vi "JSON Config With Single Term Unit Tests.vi"(8 "error in (no error)":errorcluster) -> (0 "error out":errorcluster)   [LabVIEW 2021]
uses:
  Source/Abs_Types/Double Float/Abs_Double Float.lvclass
  C:/New folder/LV_Abstract/LV_Abstract/Source/Abs_Types/Type/Abs_Type.lvclass
  Source/Abs_Types/Extended Float/Abs_Extended Float.lvclass
  Source/Abs_Types/Single Float/Abs_Single Float.lvclass
  Source/Abs_Types/Time/Abs_Time.lvclass
  Source/Abs_Types/I8 Integer/Abs_I8 Integer.lvclass
  Source/Abs_Types/I16 Integer/Abs_I16 Integer.lvclass
  Source/Abs_Types/I32 Integer/Abs_I32 Integer.lvclass
  Source/Abs_Types/I64 Integer/Abs_I64 Integer.lvclass
  Source/Abs_Types/U8 Integer/Abs_U8 Integer.lvclass
  Source/Abs_Types/U16 Integer/Abs_U16 Integer.lvclass
  Source/Abs_Types/U32 Integer/Abs_U32 Integer.lvclass
  Source/Abs_Types/U64 Integer/Abs_U64 Integer.lvclass
  Source/Abs_Types/Boolean/Abs_Boolean.lvclass
  <vilib>/numeric/Random Number (Range) DBL.vi
  bccc286b-51a7-469e-8471-aa6067be8b2c.vi
  0185a0b0-9277-4e68-a1e4-b3c67cfca5c7.vi
  39d0dc4a-455a-47ed-a8e3-229f4b41d81c.vi
  0d6305d3-07e6-45b2-bcbf-3ecd85e39c77.vi
  e5a5c62c-83b1-472a-b9f7-800ccf0aa222.vi
  cbc5ad68-3937-4771-b877-ea089d07db10.vi
  93f263c1-edcd-4840-9fac-131b8943a342.vi
  5734def3-2dae-4731-9c4b-9a8b4cb92b39.vi
  058e2dda-ae8c-4110-a64d-50d301148ec2.vi
  621c1d66-53be-4b89-8b9b-a8da23b97684.vi
  5add5537-167c-4ec9-aaa0-2258df0f0cfb.vi
  Source/Abs_Types/Abs_Simple_Read.vi
  Source/Abs_Types/Boolean/Simple Read.vi
  Source/Abs_Types/Double Float/Simple Read.vi
  Source/Abs_Types/Extended Float/Simple Read.vi
  Source/Abs_Types/Single Float/Simple Read.vi
  Source/Abs_Types/I8 Integer/Simple Read.vi
  Source/Abs_Types/I16 Integer/Simple Read.vi
  Source/Abs_Types/I32 Integer/Simple Read.vi
  Source/Abs_Types/I64 Integer/Simple Read.vi
  Source/Abs_Types/U8 Integer/Simple Read.vi
  Source/Abs_Types/U16 Integer/Simple Read.vi
  Source/Abs_Types/U32 Integer/Simple Read.vi
  Source/Abs_Types/U64 Integer/Simple Read.vi
  Source/Constants/Support/DBL/Const_DBL.lvclass
  C:/New folder/LV_Abstract/LV_Abstract/Source/Abs_Types/Double Float/Abs_Double Float.lvclass
  Source/Constants/Support/U8/Const_U8.lvclass
  C:/New folder/LV_Abstract/LV_Abstract/Source/Abs_Types/U8 Integer/Abs_U8 Integer.lvclass
  Source/Constants/Support/U16/Const_U16.lvclass
  C:/New folder/LV_Abstract/LV_Abstract/Source/Abs_Types/U16 Integer/Abs_U16 Integer.lvclass
  Source/Constants/Support/U32/Const_U32.lvclass
  C:/New folder/LV_Abstract/LV_Abstract/Source/Abs_Types/U32 Integer/Abs_U32 Integer.lvclass
  Source/Constants/Support/U64/Const_U64.lvclass
  C:/New folder/LV_Abstract/LV_Abstract/Source/Abs_Types/U64 Integer/Abs_U64 Integer.lvclass
  <vilib>/Utility/Data Type/Get Type Information.vi
  Source/Constants/Abs_Constant.vi
  Source/Constants/Support/Bool/Bool.vi
  Source/Functions/Logic/NOT.vi
  Source/Functions/Logic/Support/NOT/Bool/Method.vi
  <vilib>/addons/_JKI Toolkits/Caraya/classes/Test/Define Test.vi
  Source/Abs_Types/Type/Read Config JSON.vi
  <vilib>/addons/_JKI Toolkits/Caraya/classes/Assert/Assert.vi
  <vilib>/addons/_JKI Toolkits/Caraya/classes/Assert/Assert Equal Value_Variant.vi
  <vilib>/addons/_JKI Toolkits/Caraya/classes/Assert/Assert Equal Type_Variant.vi
  Source/Constants/Support/DBL/DBL.vi
  Source/Functions/Math/Increment.vi
  Source/Functions/Math/Support/Increment/DBL/Method.vi
  <vilib>/addons/_JKI Toolkits/Caraya/classes/Assert/Assert Almost Equal_Float.vi
  Source/Constants/Support/EXT/EXT.vi
  Source/Functions/Math/Support/Increment/EXT/Method.vi
  Source/Constants/Support/SGL/SGL.vi
  Source/Functions/Math/Support/Increment/SGL/Method.vi
  Source/Constants/Support/I8/I8.vi
  Source/Functions/Math/Support/Increment/I8/Method.vi
  Source/Constants/Support/I16/I16.vi
  Source/Functions/Math/Support/Increment/I16/Method.vi
  Source/Constants/Support/I32/I32.vi
  Source/Functions/Math/Support/Increment/I32/Method.vi
  Source/Constants/Support/I64/I64.vi
  Source/Functions/Math/Support/Increment/I64/Method.vi
  Source/Constants/Support/U8/U8.vi
  Source/Functions/Math/Support/Increment/U8/Method.vi
  Source/Constants/Support/U16/U16.vi
  Source/Functions/Math/Support/Increment/U16/Method.vi
  Source/Constants/Support/U32/U32.vi
  Source/Functions/Math/Support/Increment/U32/Method.vi
  Source/Constants/Support/U64/U64.vi
  Source/Functions/Math/Support/Increment/U64/Method.vi
  Source/Abs_Types/String/Abs_String.lvclass
  Source/Abs_Types/Complex Double Float/Abs_Complex Double Float.lvclass
  Source/Abs_Types/Complex Extended Float/Abs_Complex Extended Float.lvclass
  Source/Abs_Types/Complex Single Float/Abs_Complex Single Float.lvclass
  18c1a2b9-ea50-4f09-a971-12eb1851eb62.vi
  244b6114-7487-4987-886a-4a2847255e45.vi
  dd58c806-1dee-4031-903d-f938dbea0657.vi
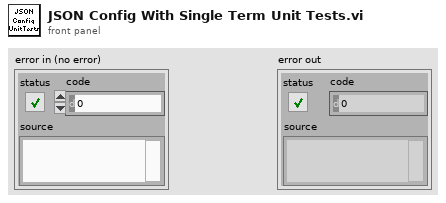
[diagram p1: front panel]
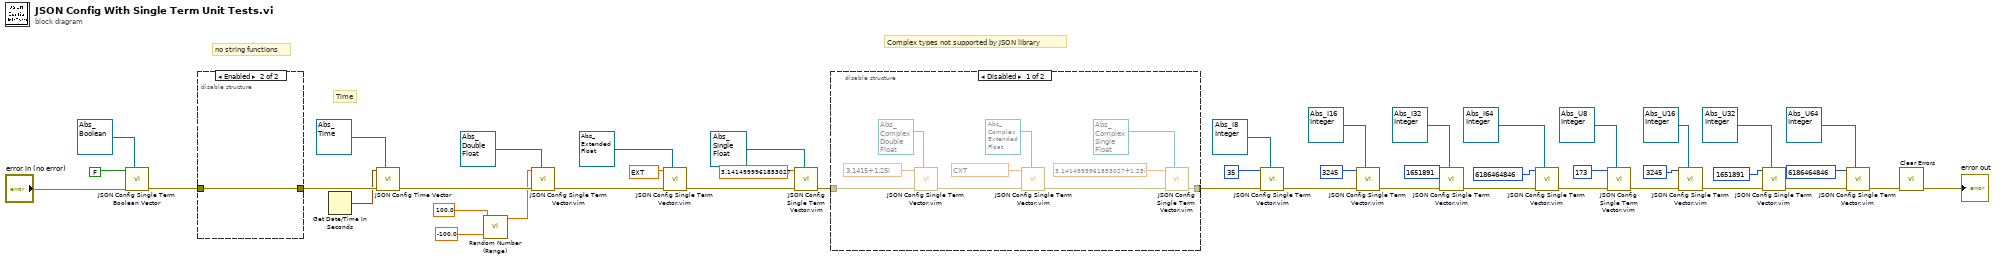
[diagram p0: block diagram]
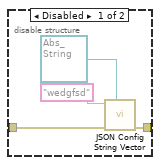
[diagram p2: hidden frame]
diagram:
  # "no string functions"
  # "Complex types not supported by JSON library"
  # "Time"
  n1 = call "JSON Config Single Term Boolean Vector.vi"("Class"=refnum<class "Abs_Boolean.lvclass"> refnum ("Abs_Boolean.lvclass"), "error in (no error)"="error in (no error)", "Test Value"=FALSE) -> ("error out"=w1:errorcluster)  [unwired: 8 in]
  n2 = disable-structure shown="Enabled" {
    disable-tunnel: [w49 w50] -> w38
    disable-tunnel: w1 -> [w46 w50]
    frame Disabled {
      n3 = call "JSON Config String Vector.vi"("Class"=refnum<class "Abs_String.lvclass"> refnum ("Abs_String.lvclass"), "error in (no error)"=w46, "Test Value"="wedgfsd") -> ("error out"=w49:errorcluster)  [unwired: 8 in]
    }
    frame Enabled {
    }
  }
  n4 = Get Date/Time In Seconds() -> (seconds since 1Jan1904=w35:timestamp)
  n5 = call "JSON Config Time Vector.vi"("Expected Class"=refnum<class "Abs_Time.lvclass"> refnum ("Abs_Time.lvclass"), "error in (no error)"=w38, "Test Value"=w35) -> ("error out"=w37:errorcluster)  [unwired: 8 in]
  n6 = call-poly <vilib>:"Random Number (Range).vi"("lower bound (0)"=-100.0, "upper bound (100)"=100.0) -> ("number"=w6:dbl)  [unwired: 9 in]
  n7 = call "JSON Config Single Term Vector.vim"("Class"=refnum<class "Abs_Double Float.lvclass"> refnum, "error in (no error)"=w37, "Test Value"=w6) -> ("error out"=w44:errorcluster)  [unwired: 8 in]
  n8 = call "JSON Config Single Term Vector.vim"("Class"=refnum<class "Abs_Extended Float.lvclass"> refnum ("Abs_Extended Float.lvclass"), "error in (no error)"=w44, "Test Value"=ext 3.1414999999999999999) -> ("error out"=w40:errorcluster)  [unwired: 8 in]
  n9 = call "JSON Config Single Term Vector.vim"("Class"=refnum<class "Abs_Single Float.lvclass"> refnum ("Abs_Single Float.lvclass"), "error in (no error)"=w40, "Test Value"=sgl 3.1415) -> ("error out"=w34:errorcluster)  [unwired: 8 in]
  n10 = disable-structure shown="Disabled" {
    disable-tunnel: w34 -> [w59 w61]
    disable-tunnel: [w51 w61] -> w33
    frame Disabled {
      n11 = call "JSON Config Single Term Vector.vim"("Class"=refnum<class "Abs_Complex Double Float.lvclass"> refnum ("Abs_Complex Double Float.lvclass"), "error in (no error)"=w59, "Test Value"=cdb 3.1415+1.25i) -> ("error out"=w56:errorcluster)  [unwired: 8 in]
      n12 = call "JSON Config Single Term Vector.vim"("Class"=refnum<class "Abs_Complex Extended Float.lvclass"> refnum ("Abs_Complex Extended Float.lvclass"), "error in (no error)"=w56, "Test Value"=cxt 3.1415+1.25i) -> ("error out"=w53:errorcluster)  [unwired: 8 in]
      n13 = call "JSON Config Single Term Vector.vim"("Class"=refnum<class "Abs_Complex Single Float.lvclass"> refnum ("Abs_Complex Single Float.lvclass"), "error in (no error)"=w53, "Test Value"=csg 3.1415+1.25i) -> ("error out"=w51:errorcluster)  [unwired: 8 in]
    }
    frame Enabled {
    }
  }
  n14 = call "JSON Config Single Term Vector.vim"("Class"=refnum<class "Abs_I8 Integer.lvclass"> refnum ("Abs_I8 Integer.lvclass"), "error in (no error)"=w33, "Test Value"=i8 35) -> ("error out"=w29:errorcluster)  [unwired: 8 in]
  n15 = call "JSON Config Single Term Vector.vim"("Class"=refnum<class "Abs_I16 Integer.lvclass"> refnum ("Abs_I16 Integer.lvclass"), "error in (no error)"=w29, "Test Value"=i16 3245) -> ("error out"=w26:errorcluster)  [unwired: 8 in]
  n16 = call "JSON Config Single Term Vector.vim"("Class"=refnum<class "Abs_I32 Integer.lvclass"> refnum ("Abs_I32 Integer.lvclass"), "error in (no error)"=w26, "Test Value"=1651891) -> ("error out"=w23:errorcluster)  [unwired: 8 in]
  n17 = call "JSON Config Single Term Vector.vim"("Class"=refnum<class "Abs_I64 Integer.lvclass"> refnum ("Abs_I64 Integer.lvclass"), "error in (no error)"=w23, "Test Value"=i64 6186464846) -> ("error out"=w20:errorcluster)  [unwired: 8 in]
  n18 = call "JSON Config Single Term Vector.vim"("Class"=refnum<class "Abs_U8 Integer.lvclass"> refnum ("Abs_U8 Integer.lvclass"), "error in (no error)"=w20, "Test Value"=u8 173) -> ("error out"=w18:errorcluster)  [unwired: 8 in]
  n19 = call "JSON Config Single Term Vector.vim"("Class"=refnum<class "Abs_U16 Integer.lvclass"> refnum ("Abs_U16 Integer.lvclass"), "error in (no error)"=w18, "Test Value"=u16 3245) -> ("error out"=w15:errorcluster)  [unwired: 8 in]
  n20 = call "JSON Config Single Term Vector.vim"("Class"=refnum<class "Abs_U32 Integer.lvclass"> refnum ("Abs_U32 Integer.lvclass"), "error in (no error)"=w15, "Test Value"=u32 1651891) -> ("error out"=w12:errorcluster)  [unwired: 8 in]
  n21 = call "JSON Config Single Term Vector.vim"("Class"=refnum<class "Abs_U64 Integer.lvclass"> refnum ("Abs_U64 Integer.lvclass"), "error in (no error)"=w12, "Test Value"=u64 6186464846) -> ("error out"=w9:errorcluster)  [unwired: 8 in]
  n22 = call <vilib>:"Clear Errors.vi"("error in (no error)"=w9) -> ("error out"=→"error out":errorcluster)  [unwired: 5 in, 1 out]
